vi "AS2.vi"() -> ()   [LabVIEW 2025]
uses:
  State.ctl
panel:
  in  "Start":bool
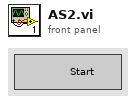
[diagram p1: front panel]
types:
  T1 = typedef "State.ctl" = enum16{"Initialize"}
  T2 = enum8{"Enabled", "Disabled", "Disabled and Grayed Out"}
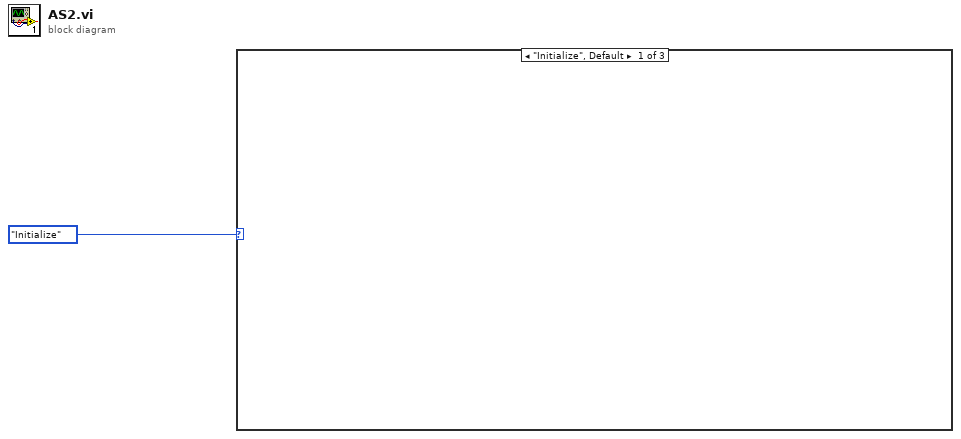
[diagram p0: block diagram]
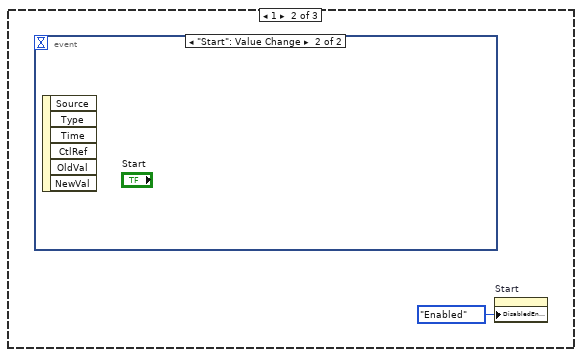
[diagram p2: hidden frame]
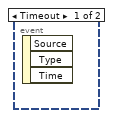
[diagram p3: hidden frame]
diagram:
  n1 = case shown="\"Initialize\", Default" State."Initialize" ("State") {
    frame "Initialize", Default {
    }
    frame 1 {
      n2 = event shown="[1] \"Start\": Value Change" {
        selector: _ -> [_ _]
        dyn-events: _ -> [_ _]
        timeout: _ -> [_ _]
        event Timeout {
          n3 = event-data() -> ()  [unwired: 1 in, 3 out]
        }
        event "Start": Value Change {
          n4 = event-data() -> ()  [unwired: 1 in, 6 out]
        }
      }
      n5 = property on="Start" class="Bool"("DisabledEnum"=T2."Enabled" ("Disabled")) -> ()  [unwired: 2 in, 2 out]
    }
    frame "Initialize" {
    }
  }
